vi "Filter Wheel Find Shortest Distance.vi"(10 "Target Filter":i32, 11 "Curr Filter":i32) -> (2 "forward?":bool, 3 "Notches":i32[](array[numeric]))   [LabVIEW 2024]
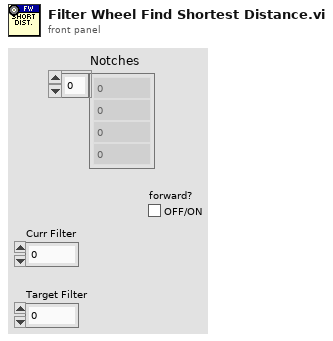
[diagram p1: front panel]
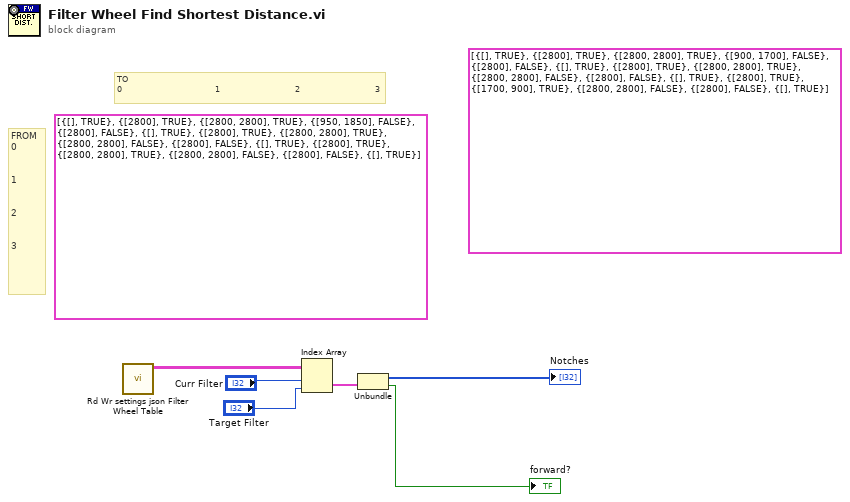
[diagram p0: block diagram]
diagram:
  (unwired) cluster{i32[], bool}[][] [[{[], TRUE}, {[2800], TRUE}, {[2800, 2800], TRUE}, {[900, 1700], FALSE}], [{[2800], FALSE}, {[], TRUE}, {[2800], TRUE}, {[2800, 2800], TRUE}], [{[2800, 2800], FALSE}, {[2800], FALSE}, {[], TRUE}, {[2800], TRUE}], [{[1700, 900], TRUE}, {[2800, 2800], FALSE}, {[2800], FALSE}, {[], TRUE}]]
  (unwired) cluster{i32[], bool}[][] [[{[], TRUE}, {[2800], TRUE}, {[2800, 2800], TRUE}, {[950, 1850], FALSE}], [{[2800], FALSE}, {[], TRUE}, {[2800], TRUE}, {[2800, 2800], TRUE}], [{[2800, 2800], FALSE}, {[2800], FALSE}, {[], TRUE}, {[2800], TRUE}], [{[2800, 2800], TRUE}, {[2800, 2800], FALSE}, {[2800], FALSE}, {[], TRUE}]]
  # "FROM\n0\n\n\n1\n\n\n2\n\n\n3"
  # "TO\n0                               1                         2                         3"
  n1 = call "Rd Wr settings json Filter Wheel Table.vi"() -> ("Filter Wheel Table"=w2:cluster{i32[], bool}[][])  [unwired: 10 in, 1 out]
  n2 = Index Array(array=w2, index (row)="Curr Filter", index (col)="Target Filter") -> (element=w6:cluster{i32[], bool})
  n3 = Unbundle(w6) -> (→"Notches":i32[], →"forward?":bool)
